vi "Get Temperature Range.vi"(8 "error in (no error)":errorcluster, 10 "maxtemp":i32, 11 "mintemp":i32) -> (0 "error out":errorcluster, 1 "function return":u32, 2 "maxtemp out":i32, 3 "mintemp out":i32)   [LabVIEW 2018, in "AndorSDK.lvlib"]
doc: "EXPNETTYPE unsigned int WINAPI GetTemperatureRange(int * mintemp, int * maxtemp);"
uses:
  AndorSDK.lvlib
  ATMCD32D.dll
  OwnVIs/AndorOWN.lvlib
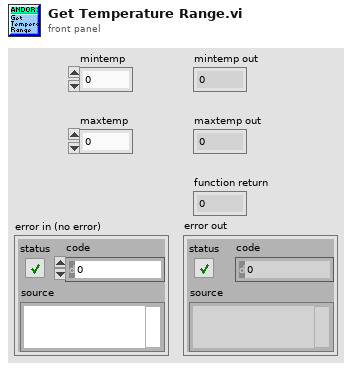
[diagram p1: front panel]
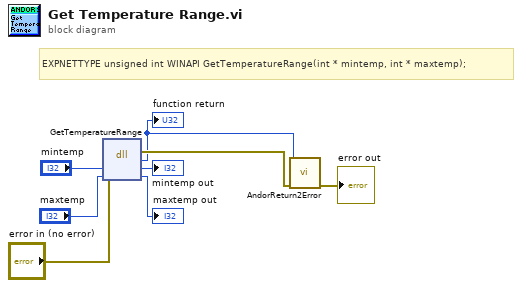
[diagram p0: block diagram]
diagram:
  # "EXPNETTYPE unsigned int WINAPI GetTemperatureRange(int * mintemp, int * maxtemp);"
  n1 = dll-call lib="C:/Users/e14user/Documents/LabVIEW software/GitRepo/lib/ANDOR/Andor SDK/ATMCD32D.*" fn="GetTemperatureRange"(error in="error in (no error)", "mintemp"="mintemp", "maxtemp"="maxtemp") -> (error out=w3:errorcluster, w2:u32, "mintemp"=→"mintemp out":i32, "maxtemp"=→"maxtemp out":i32)  [unwired: 2 in, 1 out]
  "function return" <- w2
  n2 = call "AndorReturn2Error.vi"("error in (no error)"=w3, "Camera return"=w2) -> ("error out"=→"error out":errorcluster)  [unwired: 9 in]
